vi "GetResponse.vi"(4 "error in (no error)":errorcluster, 7 "connection ID":refnum<k5>) -> (0 "error out":errorcluster, 2 "response":string, 3 "connection ID out":refnum<k5>)   [LabVIEW 2025, in "CAENels FAST-PS.lvlib"]
uses:
  CAENels FAST-PS.lvlib
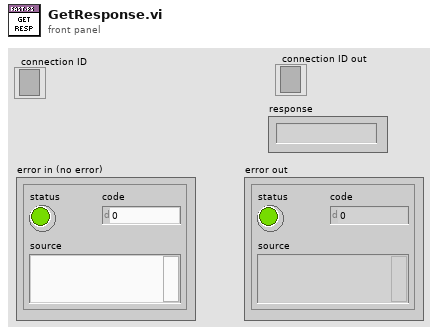
[diagram p1: front panel]
types:
  T1 = enum16{"Standard", "Buffered", "CRLF", "Immediate"}
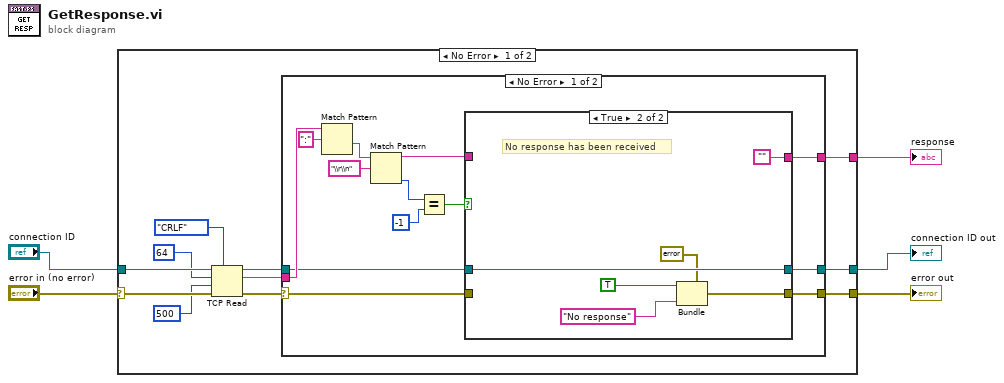
[diagram p0: block diagram]
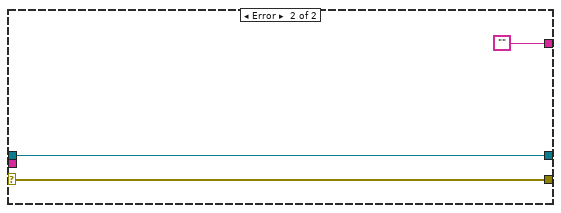
[diagram p3: hidden frame]
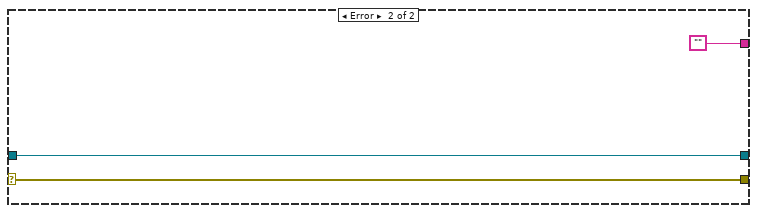
[diagram p4: hidden frame]
diagram:
  n1 = case shown="No Error" "error in (no error)" {
    selector: "error in (no error)" -> [w16 w44]
    tunnel: "connection ID" -> [w15 w43]
    tunnel: [w10 w44] -> w3
    tunnel: [w9 w43] -> w2
    tunnel: [w6 ""] -> w1
    frame No Error {
      n2 = TCP Read(connection ID=w15, bytes to read=64, error in (no error)=w16, 7:T1."CRLF" ("mode (standard)"), 9:500 ("timeout ms (25000)")) -> (connection ID out=w8:refnum<k5>, data out=w7:string, error out=w11:errorcluster)
      n3 = case shown="No Error" w11 {
        selector: w11 -> [w26 w41]
        tunnel: [w25 w41] -> w10
        tunnel: [w23 w40] -> w9
        tunnel: w8 -> [w24 w40]
        tunnel: w7 -> [w29 _]
        tunnel: [w17 ""] -> w6
        frame No Error {
          n4 = Match Pattern(string=w29, regular expression=":") -> (after substring=w21:string)  [unwired: 4 out]
          n5 = Match Pattern(string=w21, regular expression="\\r\\n") -> (before substring=w18:string, offset past match=w19:i32)  [unwired: 3 out]
          n6 = Equal?(x=w19, y=-1) -> (x = y?=w27:bool)
          n7 = case shown="True" w27 {
            tunnel: [w32 w37] -> w25
            tunnel: w26 -> [w32 _]
            tunnel: w24 -> [w31 w38]
            tunnel: [w31 w38] -> w23
            tunnel: [w30 ""] -> w17
            tunnel: w18 -> [w30 _]
            frame False {
              # "Response has been found"
            }
            frame True {
              # "No response has been received"
              n8 = Bundle(cluster=errorcluster {"status"=FALSE, "code"=0, "source"=""} ("error in  2"), "status"=TRUE, "source"="No response") -> (w37:errorcluster)  [unwired: 1 in]
            }
          }
        }
        frame Error {
        }
      }
    }
    frame Error {
    }
  }
  "error out" <- w3
  "connection ID out" <- w2
  "response" <- w1
